vi "Test Save JPG (Memory).vi"(8 "error in (no error)":errorcluster) -> (0 "error out":errorcluster, 3 "Pass?":bool)   [LabVIEW 2020]
uses:
  <vilib>/picture/picture.llb/imagedata.ctl
  G-Image/Image IO/Polymorphic VIs/Save PNG Image (Memory).vi/23d07dd8-0246-46c8-8885-479f1b0fb2b3.vi
  G-Image/Private/Result To Error.vi
  G-Image/Private/Get Image Data.vi
  G-Image/Private/ARGB To RGBA.vi
  G-Image/Private/Depth To Number Channels.vi
  G-Image/Image Processing/Indexed Color To True Color Image.vi
  <vilib>/Utility/error.llb/Error Cluster From Error Code.vi
  G-Image/Image IO/Polymorphic VIs/Load Image (Memory).vi
  G-Image/G-Image.lvlib
  G-Image/Image IO/Polymorphic VIs/Save JPG Image (Memory).vi
panel:
  out "Array":cluster{string, "new picture":picture}[](array[cluster])
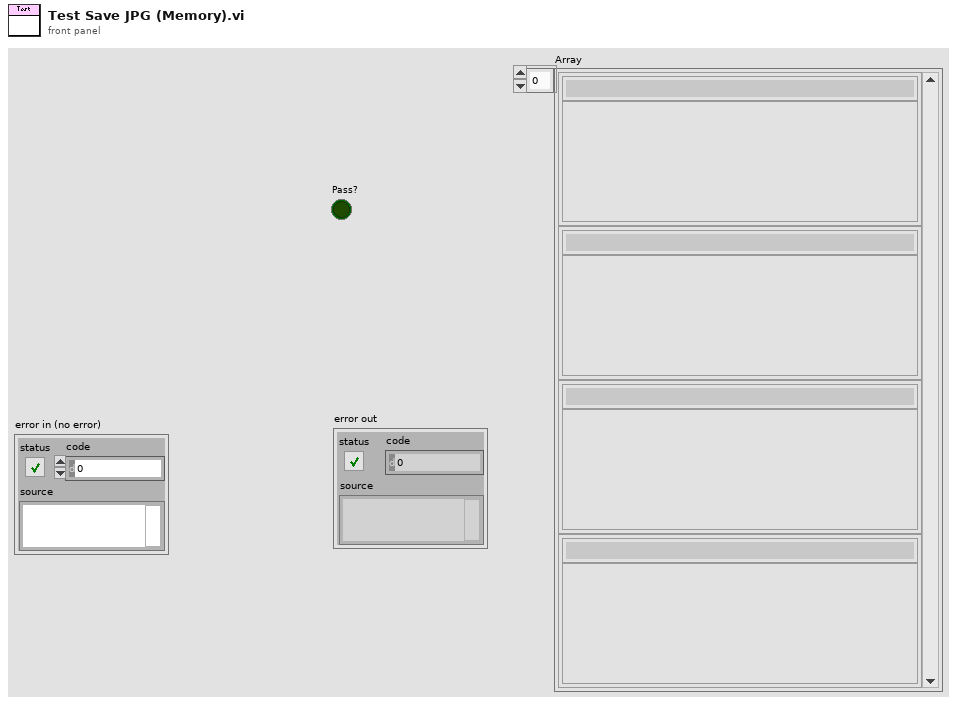
[diagram p1: front panel]
types:
  T1 = typedef "imagedata.ctl" = cluster{"image type":i32, "image depth":i32, "image":u8[], "mask":u8[], "colors":u32[], "Rectangle":cluster{"left":i16, "top":i16, "right":i16, "bottom":i16}}
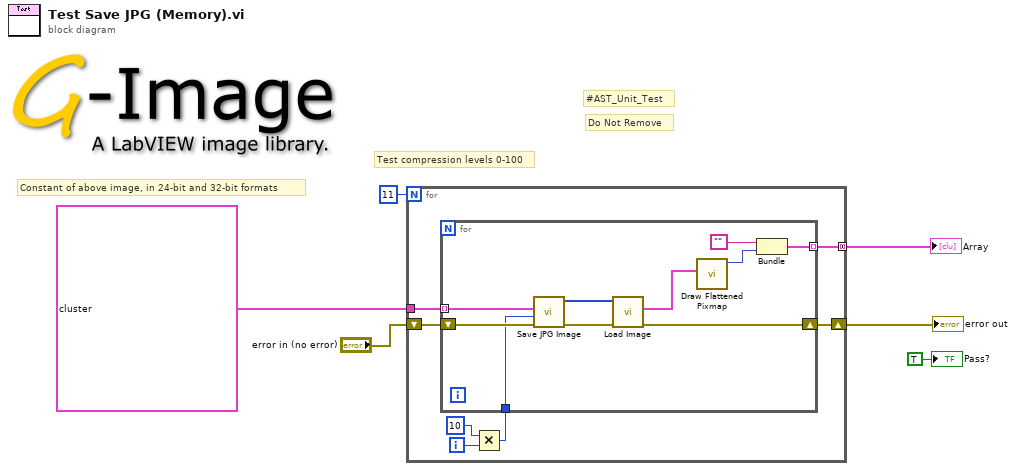
[diagram p0: block diagram]
diagram:
  # "Test compression levels 0-100"
  # "Constant of above image, in 24-bit and 32-bit formats"
  # "Do Not Remove"
  # "#AST_Unit_Test"
  n1 = for {
    N: 11 -> [_]
    tunnel: [w12] -> w5 mode=concatenating
    tunnel: T1[] [{"image type"=0, "image depth"=24, "image"=array[115500 elements], "mask"=[], "colors"=[], "Rectangle"={"left"=0, "top"=0, "right"=350, "bottom"=110}}, {"image type"=0, "image depth"=32, "image"=array[154000 elements], "mask"=array[4840 elements], "colors"=[], "Rectangle"={"left"=0, "top"=0, "right"=350, "bottom"=110}}] ("Array 2") -> [w10]
    shift-right: [w11] -> w4
    shift-left: "error in (no error)" -> [w13]
    i -> [w9]
    n2 = Multiply(x=10, y=w9) -> (x*y=w7:i32)
    n3 = for {
      tunnel: w10 -> [w20] mode=indexing
      shift-right: [w14] -> w11
      shift-left: w13 -> [w23]
      tunnel: [w17] -> w12 mode=indexing
      tunnel: w7 -> [w16]
      n4 = call-poly "Save JPG Image.vi"("error in (no error)"=w23, "Quality (85)"=w16, "Image"=w20) -> ("error out"=w21:errorcluster, "Encoded Image"=w22:u8[])  [unwired: 7 in]
      n5 = call-poly "Load Image.vi"("error in (no error)"=w21, "Encoded Image"=w22) -> ("error out"=w14:errorcluster, "Image"=w19:T1)  [unwired: 8 in]
      n6 = call <vilib>:"Draw Flattened Pixmap.vi"("image data"=w19) -> ("new picture"=w18:picture)  [unwired: 8 in]
      n7 = Bundle("", "new picture"=w18) -> (w17:cluster{string, "new picture":picture})  [unwired: 1 in]
    }
  }
  "error out" <- w4
  "Array" <- w5
  "Pass?" <- TRUE ("Pass?")
